vi "scaleFeaturesPositions_XY_um_pix.vi"(8 "error in (no error)":errorcluster, 11 "?":T1={"PythonSession"=refnum, "PythonOpen?"=FALSE, "State"=enum."WAIT", "Display"=FALSE, "Holo parameters"={"wavelength"=6.6e-07, "optical index"=1.33, "Holo size X"=1024, "Holo size Y"=1024, "pixel size"=7e-06, "objective magnification"=40.0}, "BinThreshold"=0.0, "HOLOGRAM PATH"=path "C:/TRAVAIL/developpement/imagesHolo/20um_bon_40X/20um_40x_int_.7ajp1c6t.000000.bmp", "HOLOGRAM DIRECTORY"=path "C:/TRAVAIL/developpement/imagesHolo/20um_bon_40X/20um_40x_int_.7ajp1c6t.000000.bmp", "LIST HOLO BATCH"=[], "Display"=[], "meanHolo"=[], "FEATURES(µm)"=[], "LabelPicture"="", "Status"="", "planeToDisplayFeatures"=enum."XY", "Analyse parameters"={"propagation"={"distance ini"=0.0, "number of planes"=100, "step"=1e-06, "Fourier BP filter (pix)"={"High pass (0=none)"=15.0, "Low Pass (0=none)"=125.0}}, "Focus"={"Type"=enum."TENENGRAD", "Sum size"=20}, "Remove mean Hologram"=FALSE, "CCL parameters"={"Threshold ( N x Standard deviation)"=10.0, "Connectivity"=enum."26", "min voxel"=1.0, "max voxel"=0.0}}} {"Analyse parameters"."CCL parameters"."max voxel" min=0.0 max=0.0; "Analyse parameters"."CCL parameters"."min voxel" min=1.0 max=100.0; "Analyse parameters"."CCL parameters"."Threshold ( N x Standard deviation)" min=1.0 max=100.0; "Analyse parameters"."Focus"."Sum size" min=1 max=100; "Analyse parameters"."propagation"."Fourier BP filter (pix)"."Low Pass (0=none)" format="%#_6e"; "Analyse parameters"."propagation"."step" format="%#_6e"; "Analyse parameters"."propagation"."distance ini" format="%#_6e"; "Holo parameters"."wavelength" format="%#_6e"}) -> (0 "error out":errorcluster, 3 "XYFeatures(pix)":sgl[][](array[numeric]))   [LabVIEW 2023, in "holoPyTracks.lvlib"]
uses:
  HoloPyLib/holoPyTracks.lvlib
  HologramInfo.ctl
  HoloPyLib/CCL_parameters.ctl
  datas.ctl
  analyse_parameters.ctl
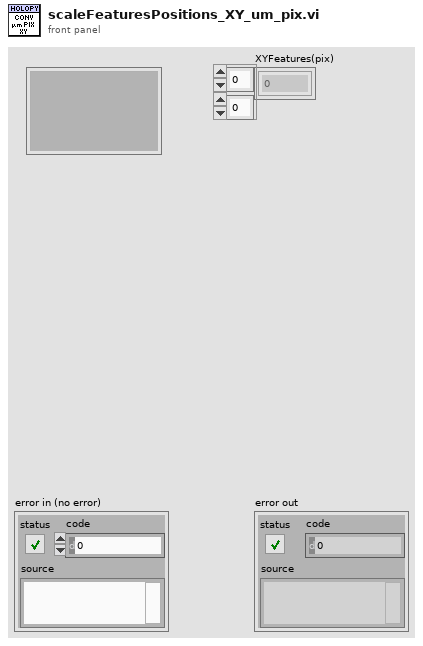
[diagram p1: front panel]
types:
  T1 = typedef "datas.ctl" = cluster{"PythonSession":refnum<k35>, "PythonOpen?":bool, "State":enum16{"WAIT", "TEST", "BATCH"}, "Display":bool, "Holo parameters":T2, "BinThreshold":sgl, "HOLOGRAM PATH":path, "HOLOGRAM DIRECTORY":path, "LIST HOLO BATCH":path[], "Display":sgl[][], "meanHolo":sgl[][], "FEATURES(µm)":sgl[][], "LabelPicture":string, "Status":string, "planeToDisplayFeatures":enum16{"XY", "XZ", "YZ"}, "Analyse parameters":T3}
  T2 = typedef "holoPyTracks.lvlib/HologramInfo.ctl" = cluster{"wavelength":sgl, "optical index":sgl, "Holo size X":i32, "Holo size Y":i32, "pixel size":sgl, "objective magnification":sgl}
  T3 = typedef "holoPyTracks.lvlib/analyse_parameters.ctl" = cluster{"propagation":cluster{"distance ini":dbl, "number of planes":i32, "step":dbl, "Fourier BP filter (pix)":cluster{"High pass (0=none)":dbl, "Low Pass (0=none)":dbl}}, "Focus":cluster{"Type":enum16{"SUM_OF_INTENSITY", "SUM_OF_LAPLACIAN", "SUM_OF_VARIANCE", "TENENGRAD"}, "Sum size":i32}, "Remove mean Hologram":bool, "CCL parameters":T4}
  T4 = typedef "CCL_parameters.ctl" = cluster{"Threshold ( N x Standard deviation)":dbl, "Connectivity":enum16{"6", "18", "26"}, "min voxel":dbl, "max voxel":dbl}
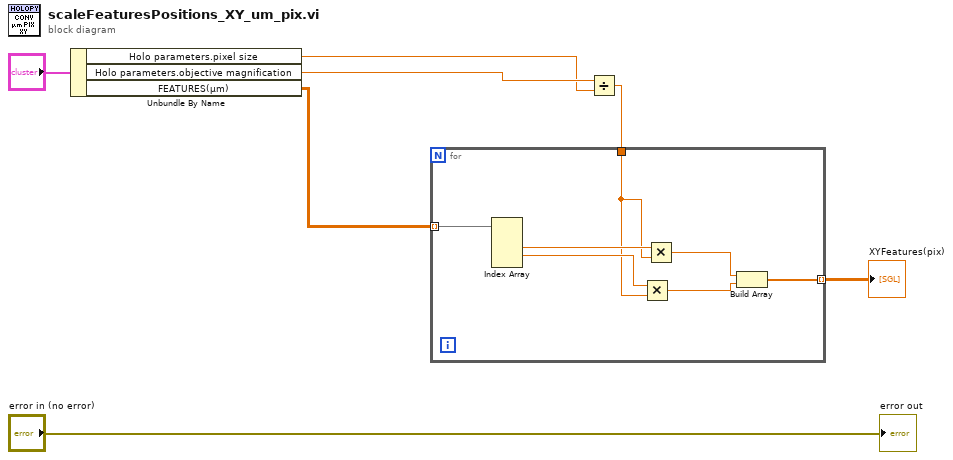
[diagram p0: block diagram]
diagram:
  n1 = Unbundle By Name("?") -> ("Holo parameters.pixel size"=w6:sgl, "Holo parameters.objective magnification"=w7:sgl, "FEATURES(µm)"=w1:sgl[][])
  n2 = Divide(x=w7, y=w6) -> (x/y=w5:sgl)
  n3 = for {
    tunnel: w1 -> [w14] mode=indexing
    tunnel: w5 -> [w11]
    tunnel: [w8] -> w4 mode=indexing
    n4 = Index Array(array=w14) -> (element #2=w13:sgl, element #3=w12:sgl)  [unwired: 4 in, 2 out]
    n5 = Multiply(x=w12, y=w11) -> (x*y=w9:sgl)
    n6 = Multiply(x=w13, y=w11) -> (x*y=w10:sgl)
    n7 = Build Array(w10, w9) -> (w8:sgl[])
  }
  "XYFeatures(pix)" <- w4
  "error out" <- "error in (no error)"
